vi "RD Analog In Read.vi"(0 "handle":u64, 5 "ch":i32, 7 "size":i32, 9 "range":dbl, 11 "error in (no error)":errorcluster caption="错误输入（无错误）", 12 "CalArray":u8[](array[numeric])) -> (3 "RxBuffer out":dbl[](array[numeric]), 4 "handle out":u64, 6 "backsize out":i32, 8 "function return":i32, 14 "CalArray out":u8[](array[numeric]), 15 "error out":errorcluster caption="错误输出")   [LabVIEW 2018, in "InstrumentsPlayground.lvlib"]
doc: "CLIFFAPI int CliffAnalogInRead(FT_HANDLE handle,int ch, int size,double range, double *RxBuffer,int* CalArray,int *backsize);"
uses:
  InstrumentsPlayground.lvlib
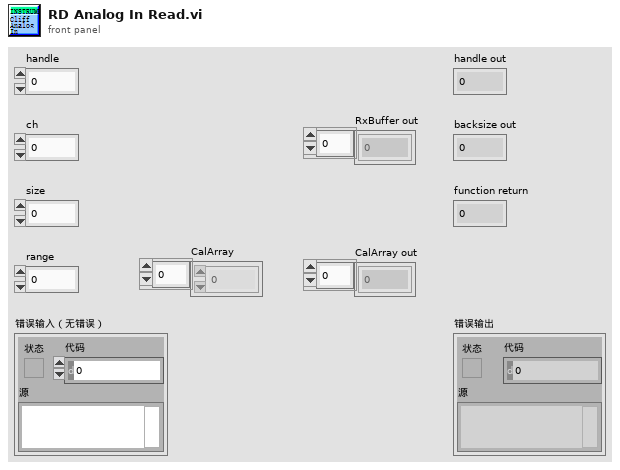
[diagram p1: front panel]
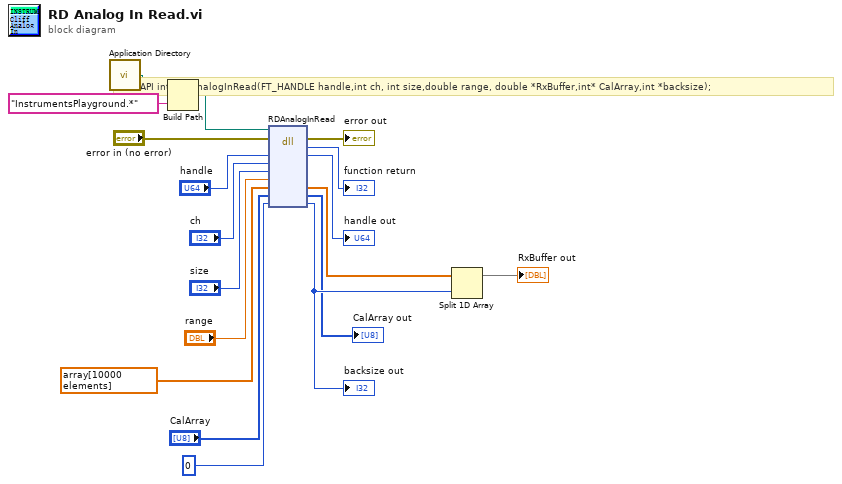
[diagram p0: block diagram]
diagram:
  # "CLIFFAPI int CliffAnalogInRead(FT_HANDLE handle,int ch, int size,double range, double *RxBuffer,int* CalArray,int *backsize);"
  n1 = call <vilib>:"Application Directory.vi"() -> ("Application Directory"=w7:path)
  n2 = Build Path(base path=w7, name or relative path="InstrumentsPlayground.*" ("名称或相对路径")) -> (appended path=w6:path)
  n3 = dll-call lib="E:/Work/YZCourse_Xtext/Cliff/API/IPLabView lib/InstrumentsPlayground.*" fn="RDAnalogInRead"(path in=w6, error in="error in (no error)", "handle"="handle", "ch"="ch", "size"="size", "range"="range", "RxBuffer"=dbl[] array[10000 elements], "CalArray"="CalArray", "backsize"=0) -> (error out=→"error out":errorcluster, "返回类型"=→"function return":i32, "handle"=→"handle out":u32, "RxBuffer"=w5:dbl[], "CalArray"=→"CalArray out":u8[], "backsize"=w3:i32)  [unwired: 4 in, 1 out]
  "backsize out" <- w3
  n4 = Split 1D Array(array=w5, index=w3) -> (first subarray=→"RxBuffer out":dbl[])  [unwired: 1 out]
